vi "Unregister.vi"(8 "Error In":errorcluster, 10 "Registrant Enq":refnum<class "Message Enqueuer.lvclass">, 11 "Event Source In":refnum<class "Event Source Actor.lvclass">) -> (0 "Error Out":errorcluster, 3 "Event Source Out":refnum<class "Event Source Actor.lvclass">)   [LabVIEW 2020, in "Event Source.lvlib" / "Event Source Actor.lvclass"]
doc: "This method unregisters a specific Actors Enqueuer from all Events he is listening to from this Event Source Actor."
uses:
  Event Source Actor.lvclass
  <vilib>/ActorFramework/Message Enqueuer/Message Enqueuer.lvclass
  Event Source Actor.lvclass/Event Source Actor.ctl
  48172011-38dd-4e95-b88c-c50fd512a03c.vi
  Program Files/National Instruments/LabVIEW 2020/resource/AFDebug/AF Debug.lvlib
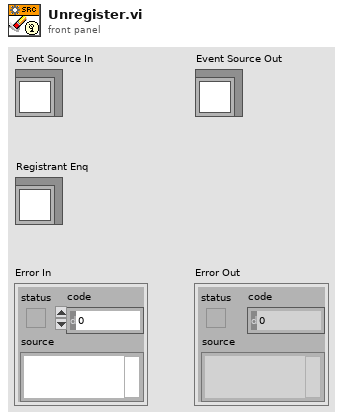
[diagram p1: front panel]
types:
  T1 = map{string, set{refnum<class "Message Enqueuer.lvclass">}}
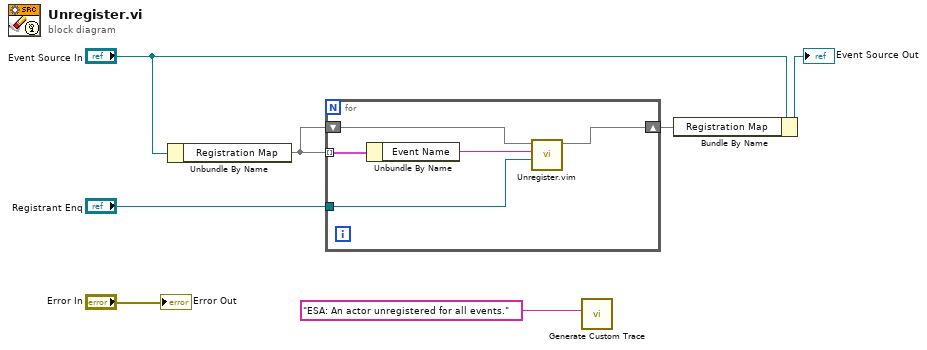
[diagram p0: block diagram]
diagram:
  n1 = Unbundle By Name("Event Source In") -> ("Registration Map"=w7:T1)
  n2 = for {
    tunnel: w7 -> [w12] mode=indexing
    shift-right: [w8] -> w5
    shift-left: w7 -> [w10]
    tunnel: "Registrant Enq" -> [w9]
    n3 = Unbundle By Name(w12) -> ("Event Name"=w11:string)
    n4 = call "Unregister.vim"("set element"=w9, "key"=w11, "map in"=w10) -> ("map out"=w8:T1)  [unwired: 6 in, 2 out]
  }
  n5 = call "Generate Custom Trace.vi"("Custom Action"="ESA: An actor unregistered for all events.") -> ()  [unwired: 11 in]
  n6 = Bundle By Name(cluster="Event Source In", "Registration Map"=w5) -> (→"Event Source Out":refnum<class "Event Source Actor.lvclass">)
  "Error Out" <- "Error In"
